vi "Write Default AppBar Actor.vi"(8 "error in (no error)":errorcluster, 10 "Win8uiFramework.lvlib:ViewableActor.lvclass":refnum<class "ViewableActor.lvclass">, 11 "MainController in":refnum<class "MainController.lvclass">) -> (0 "error out":errorcluster, 3 "MainController out":refnum<class "MainController.lvclass">)   [LabVIEW 2012, in "Win8uiFramework.lvlib" / "MainController.lvclass"]
uses:
  MainController.lvclass
  ViewableActor.lvclass
  MainController.lvclass/MainController.ctl
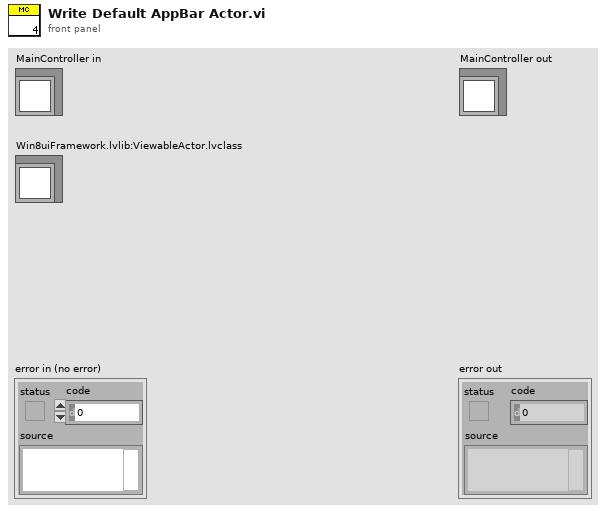
[diagram p1: front panel]
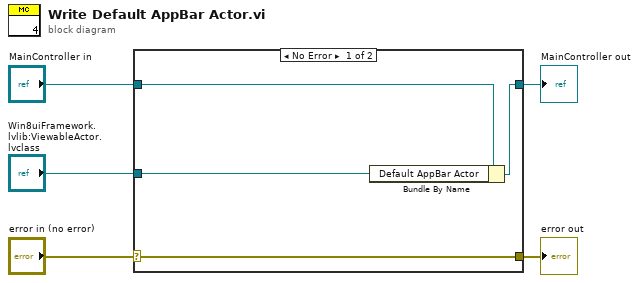
[diagram p0: block diagram]
diagram:
  n1 = case shown="No Error" "error in (no error)" {
    selector: "error in (no error)" -> [w9 w10]
    tunnel: [w9 w10] -> w4
    tunnel: [w7 w11] -> w2
    tunnel: "MainController in" -> [w8 w11]
    tunnel: "Win8uiFramework.lvlib:ViewableActor.lvclass" -> [w6 _]
    frame No Error {
      n2 = Bundle By Name(cluster=w8, "Default AppBar Actor"=w6) -> (w7:refnum<class "MainController.lvclass">)
    }
    frame Error {
    }
  }
  "error out" <- w4
  "MainController out" <- w2
